vi "追溯Global.vi"() -> ()   [LabVIEW 2020]
panel:
  out "CODEMAIN_ID":string
  out "PRESEN_ID":string
  in  "字符串 2":string
  in  "字符串":string
  out "PREMAIN_ID":string
  out "DEVICE_ID":string
  out "USER_ID":string
  out "PRODUCT_ID":string
  out "CODESEN_ID":string
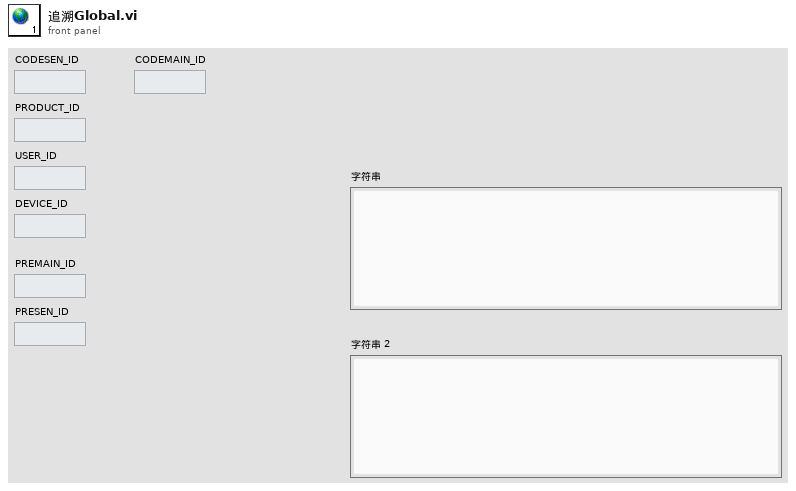
[diagram p1: front panel]
diagram:
